vi "Write ILC.vi"(10 "ILC":refnum<class "ILC.lvclass">, 11 "ILCDAC4 in":refnum<class "ILCDAC4.lvclass">) -> (3 "ILCDAC4 out":refnum<class "ILCDAC4.lvclass">)   [LabVIEW 2015]
uses:
  ILCDAC4.lvclass
  <userlib>/Common/ILC/ILC/ILC.lvclass
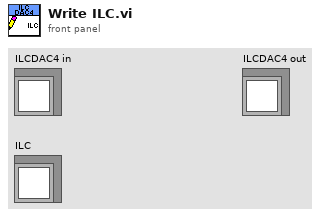
[diagram p1: front panel]
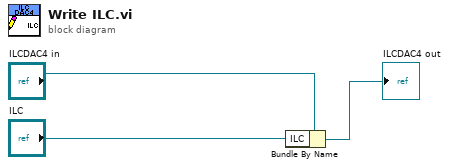
[diagram p0: block diagram]
diagram:
  n1 = Bundle By Name(cluster="ILCDAC4 in", "ILC"="ILC") -> (→"ILCDAC4 out":refnum<class "ILCDAC4.lvclass">)
